vi "Read and Update Metadata.vi"(8 "error in (no error)":errorcluster, 11 "Update Metadata":bool) -> (0 "error out":errorcluster, 3 "Plugin Info":T1[](array[typedef]))   [LabVIEW 2021, in "CIFPluginLoader.lvclass"]
uses:
  CIFPluginLoader.lvclass
  CIFPluginLoader.lvclass/CIFPluginLoader.ctl
  CIFUtilities/CIFConfigurationFile/typedef/Location Type.ctl
  CIFUtilities/CIFConfigurationFile/CIF Configuration File.lvlib
  <vilib>/Utility/config.llb/NI_LVConfig.lvlib
  CIFCore/Common/Typedef/Version.ctl
  CIFCore/Common/CIFCoreCommon.lvlib
  CIFPluginManager/typedef/Plugin Metadata.ctl
  CIFPluginManager/CIFPluginManager.lvclass
  CIFPluginManager/typedef/Loader Type.ctl
  CIFPluginManager/typedef/Discovered Plugin.ctl
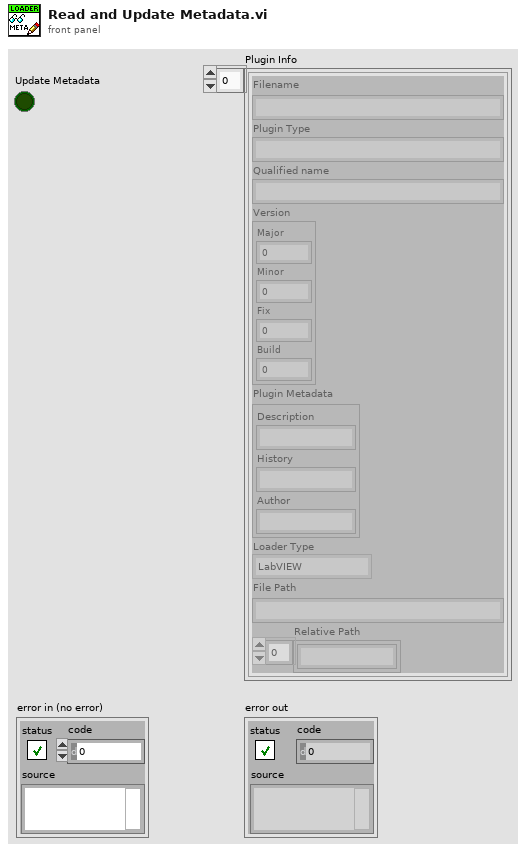
[diagram p1: front panel]
types:
  T1 = typedef "CIFPluginManager.lvclass/Discovered Plugin.ctl" = cluster{"Filename":string, "Plugin Type":string, "Qualified name":string, "Version":T2, "Plugin Metadata":T3, "Loader Type":T4, "File Path":string, "Relative Path":string[]}
  T2 = typedef "CIFCoreCommon.lvlib/Version.ctl" = cluster{"Major":i32, "Minor":i32, "Fix":i32, "Build":i32}
  T3 = typedef "CIFPluginManager.lvclass/Plugin Metadata.ctl" = cluster{"Description":string, "History":string, "Author":string}
  T4 = typedef "CIFPluginManager.lvclass/Loader Type.ctl" = enum16{"LabVIEW"}
  T5 = typedef "CIF Configuration File.lvlib/Location Type.ctl" = enum16{"Config File", "Manager", "Protos", "Plugins", "UI Plugins", "Logs", "Orchestrations", "Loaders"}
  T6 = typedef "NI_LVConfig.lvlib/Config Data RefNum.ctl" = refnum<k1>
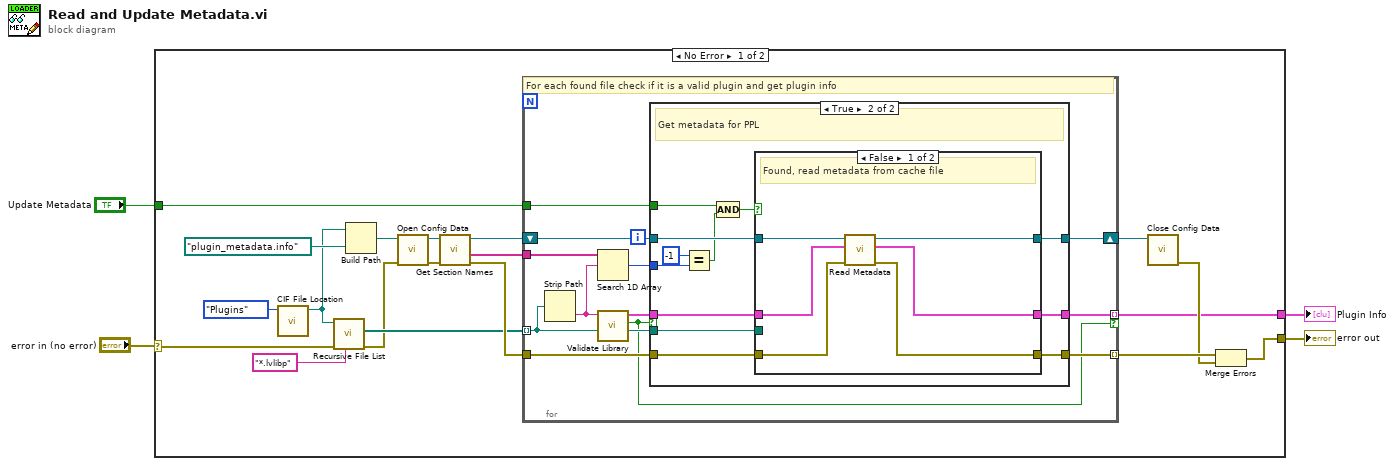
[diagram p0: block diagram]
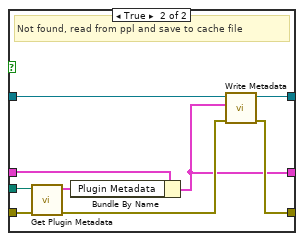
[diagram p3: hidden frame]
diagram:
  n1 = case shown="No Error" "error in (no error)" {
    selector: "error in (no error)" -> [w7 w67]
    tunnel: [w12 w67] -> w4
    tunnel: "Update Metadata" -> [w11 _]
    tunnel: [w5 _] -> w1
    frame No Error {
      n2 = call "CIF File Location.vi"("LocationType"=Location_Type."Plugins") -> ("Location"=w10:path)  [unwired: 10 in]
      n3 = call <vilib>:"Recursive File List.vi"("pattern"="*.lvlibp", "error in (no error)"=w7, "Folder Path"=w10) -> ("error out"=w6:errorcluster, "All Files in Dir"=w8:path[])  [unwired: 4 in, 3 out]
      n4 = Build Path(base path=w10, name or relative path=path "plugin_metadata.info") -> (appended path=w22:path)
      n5 = call <vilib>:"Open Config Data.vi"("error in (no error)"=w6, "configuration file path"=w22) -> ("error out"=w18:errorcluster, "refnum"=w19:T6)  [unwired: 7 in, 1 out]
      n6 = call <vilib>:"Get Section Names.vi"("error in (no error)"=w18, "refnum"=w19) -> ("error out"=w16:errorcluster, "section names"=w15:string[], "refnum out"=w17:T6)  [unwired: 7 in]
      n7 = for {
        tunnel: [w26] -> w5 mode=indexing if=w28
        tunnel: w16 -> [w36]
        tunnel: [w35] -> w14 mode=indexing
        shift-right: [w33] -> w20
        shift-left: w17 -> [w34]
        tunnel: w15 -> [w32]
        tunnel: w11 -> [w27]
        tunnel: w8 -> [w25] mode=indexing
        # "For each found file check if it is a valid plugin and get plugin info"
        n8 = Strip Path(path=w25) -> (name=w24:string)  [unwired: 1 out]
        n9 = Search 1D Array(1D array=w32, element=w24) -> (index of element=w30:i32)  [unwired: 1 in]
        n10 = call "Validate Library.vi"("path in"=w25, "Filename"=w24) -> ("path (dup)"=w29:path, "valid"=w28:bool, "Discovered Plugin"=w31:T1)  [unwired: 7 in]
        n11 = case shown="True" w28 {
          tunnel: w31 -> [w38 w41]
          tunnel: w29 -> [_ w51]
          tunnel: w36 -> [w39 w50]
          tunnel: [w38 w40] -> w26
          tunnel: [w39 w47] -> w35
          tunnel: w34 -> [w37 w49]
          tunnel: [w37 w48] -> w33
          tunnel: w30 -> [_ w46]
          tunnel: w27 -> [_ w44]
          frame False {
            # "Invalid"
          }
          frame True {
            # "Get metadata for PPL"
            n12 = Equal?(x=-1, y=w46) -> (x = y?=w43:bool)
            n13 = Compound Arithmetic op=AND(w44, w43) -> (w42:bool)
            n14 = case shown="False" w42 {
              tunnel: w41 -> [w56 w58]
              tunnel: w51 -> [_ w66]
              tunnel: w50 -> [w53 w64]
              tunnel: w49 -> [w57 w63]
              tunnel: [w54 w62] -> w48
              tunnel: [w55 w59] -> w40
              tunnel: [w52 w60] -> w47
              frame False {
                # "Found, read metadata from cache file"
                n15 = call "Read Metadata.vi"("error in (no error)"=w53, "Plugin Info in"=w56, "metadata ref in"=w57) -> ("error out"=w52:errorcluster, "Plugin Info out"=w55:T1, "metadata ref dup"=w54:T6)  [unwired: 6 in]
              }
              frame True {
                # "Not found, read from ppl and save to cache file"
                n16 = call "Get Plugin Metadata.vi"("error in (no error)"=w64, "Packed Library Path"=w66) -> ("error out"=w61:errorcluster, "Plugin Metadata"=w65:T3)  [unwired: 8 in]
                n17 = Bundle By Name(cluster=w58, "Plugin Metadata"=w65) -> (w59:T1)
                n18 = call "Write Metadata.vi"("error in (no error)"=w61, "Plugin Info"=w59, "metadata ref in"=w63) -> ("error out"=w60:errorcluster, "metadata ref dup"=w62:T6)  [unwired: 7 in]
              }
            }
          }
        }
      }
      n19 = call <vilib>:"Close Config Data.vi"("refnum"=w20) -> ("error out"=w13:errorcluster)  [unwired: 9 in, 1 out]
      n20 = Merge Errors(w14, w13) -> (w12:errorcluster)
    }
    frame Error {
    }
  }
  "error out" <- w4
  "Plugin Info" <- w1
